vi "FetchAllDbl.vi"(8 "error in (no error)":errorcluster, 11 "NiDaqMx in":refnum<class "NiDaqMx.lvclass">) -> (0 "error out":errorcluster, 3 "NiDaqMx out":refnum<class "NiDaqMx.lvclass">)   [LabVIEW 2018, in "DigitizerPlugins.lvlib" / "NiDaqMx.lvclass"]
uses:
  NiDaqMx.lvclass
  F:/Projects/ICDAS/NistPluggableModules/Digitizer/DigitizerPlugins/DigitizerBaseClass/DigitizerBase.lvclass
  DigitizerBaseClass/DigitizerBase.lvclass/DigitizerBase.ctl
  NiDaqMx.lvclass/NiDaqMx.ctl
  DigitizerBaseClass/Typedefs/WfrmAttributes.ctl
  Accessors/Write Started.vi
  <vilib>/DAQmx/read.llb/DAQmx Read (Analog 1D Wfm NChan NSamp).vi
  DigitizerBaseClass/Accessors/Read Waveforms.vi
  DigitizerBaseClass/Accessors/Write InstRef.vi
  DigitizerBaseClass/Accessors/Write Waveforms.vi
  DigitizerBaseClass/Accessors/Read InstRef.vi
  Accessors/Read Started.vi
  DigitizerBaseClass/Accessors/Read Acquisition.vi
  DigitizerBaseClass/Accessors/Read SyncInfo.vi
  Accessors/Read TsQue.vi
  <vilib>/DAQmx/miscellaneous.llb/DAQmx Fill In Error Info.vi
  DigitizerBaseClass/DigitizerBase.lvclass
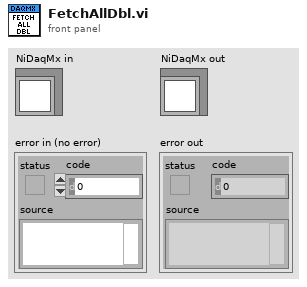
[diagram p1: front panel]
types:
  T1 = typedef "DigitizerPlugins.lvlib/DigitizerBase.lvclass/WfrmAttributes.ctl" = cluster{"XOffset":dbl, "ActualPts":i64, "FirstValid":i64}
  T2 = typedef "DigitizerPlugins.lvlib/DigitizerBase.lvclass/Acquisition.ctl" = cluster{"SampleRate":dbl, "RecordSize":i32, "NumRecords":i32, "SampleMode":i32, "Timeout (ms)":i32}
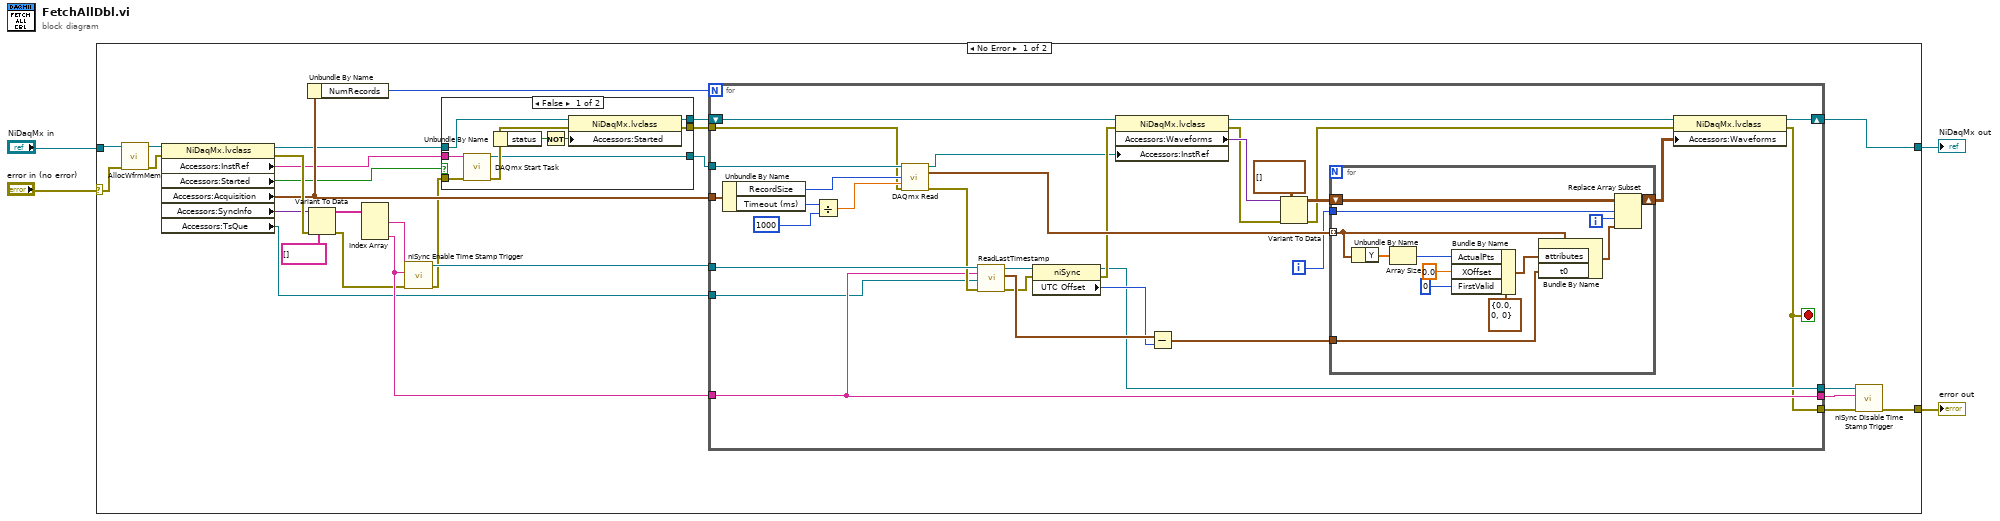
[diagram p0: block diagram]
diagram:
  n1 = case shown="No Error" "error in (no error)" {
    selector: "error in (no error)" -> [w30 w89]
    tunnel: [w15 w89] -> w3
    tunnel: [w31 w88] -> w1
    tunnel: "NiDaqMx in" -> [w29 w88]
    frame No Error {
      n2 = call-dynamic "AllocWfrmMem.vi"("error in (no error)"=w30, "DigitizerBase in"=w29) -> ("error out"=w27:errorcluster, "DigitizerBase out"=w28:refnum<class "NiDaqMx.lvclass">)  [unwired: 8 in]
      n3 = property class="NiDaqMx.lvclass"(reference=w28, error in=w27) -> (reference out=w10:refnum<class "NiDaqMx.lvclass">, error out=w25:errorcluster, "Accessors:InstRef"=w7:string, "Accessors:Started"=w8:bool, "Accessors:Acquisition"=w12:T2, "Accessors:SyncInfo"=w13:variant, "Accessors:TsQue"=w14:refnum<queue>)
      n4 = Unbundle By Name(w12) -> ("NumRecords"=w26:i32)
      n5 = Variant To Data(error in=w25, type=string[] [], Variant=w13) -> (data=w23:string[], error out=w19:errorcluster)
      n6 = Index Array(array=w23) -> (element #1=w21:string, element #3=w20:string)  [unwired: 3 in, 1 out]
      n7 = call <instrlib>:"niSync Enable Time Stamp Trigger.vi"("error in (no error)"=w19, "terminal"=w20, "instrument handle"=w21) -> ("error out"=w11:errorcluster, "instrument handle out"=w22:refnum<k15>)  [unwired: 6 in]
      n8 = case shown="False" w8 {
        tunnel: w11 -> [w40 w42]
        tunnel: w10 -> [w39 w43]
        tunnel: [w35 w43] -> w9
        tunnel: [w34 w42] -> w5
        tunnel: w7 -> [w33 w41]
        tunnel: [w32 w41] -> w6
        frame False {
          n9 = call <vilib>:"DAQmx Start Task.vi"("task/channels in"=w33, "error in"=w40) -> ("task out"=w32:refnum<k21>, "error out"=w36:errorcluster)  [unwired: 12 in]
          n10 = Unbundle By Name(w36) -> ("status"=w38:bool)
          n11 = Not(x=w38) -> (.not. x?=w37:bool)
          n12 = property class="NiDaqMx.lvclass"(reference=w39, error in=w36, "Accessors:Started"=w37) -> (reference out=w35:refnum<class "NiDaqMx.lvclass">, error out=w34:errorcluster)
        }
        frame True {
        }
      }
      n13 = for {
        N: w26 -> [_]
        tunnel: w6 -> [w72]
        tunnel: w12 -> [w66]
        shift-right: [w67] -> w31
        shift-left: w9 -> [w68]
        tunnel: w22 -> [w57]
        tunnel: w20 -> [w49]
        tunnel: [w49] -> w17
        tunnel: [w48] -> w18
        tunnel: [w47] -> w16
        tunnel: w14 -> [w46]
        tunnel: w5 -> [w45]
        i -> [w60]
        stop <- w47 stop-if-true
        n14 = Unbundle By Name(w66) -> ("RecordSize"=w71:i32, "Timeout (ms)"=w74:i32)
        n15 = Divide(x=w74, y=1000) -> (x/y=w70:dbl)
        n16 = call-poly <vilib>:"DAQmx Read.vi"("task/channels in"=w72, "number of samples per channel"=w71, "timeout"=w70, "error in"=w45) -> ("task out"=w44:refnum<k21>, "data"=w69:waveform(dbl)[], "error out"=w56:errorcluster)  [unwired: 9 in]
        n17 = call "ReadLastTimestamp.vi"("error in (no error)"=w56, "TsQue"=w46, "Terminal"=w49, "instrument handle"=w57) -> ("error out"=w51:errorcluster, "time stamp out"=w55:timestamp, "instrument handle out"=w52:refnum<k15>)  [unwired: 5 in]
        n18 = property class="niSync"(reference=w52, error in=w51) -> (reference out=w48:refnum<k15>, error out=w50:errorcluster, "UTC Offset"=w54:i32)
        n19 = property class="NiDaqMx.lvclass"(reference=w68, error in=w50, "Accessors:InstRef"=w44) -> (reference out=w65:refnum<class "NiDaqMx.lvclass">, error out=w62:errorcluster, "Accessors:Waveforms"=w63:variant)
        n20 = Subtract(x=w55, y=w54) -> (x-y=w53:timestamp)
        n21 = Variant To Data(error in=w62, type=waveform(dbl)[][] [], Variant=w63) -> (data=w61:waveform(dbl)[][], error out=w59:errorcluster)
        n22 = for {
          tunnel: w69 -> [w85] mode=indexing
          shift-right: [w79] -> w58
          shift-left: w61 -> [w80]
          tunnel: w60 -> [w76]
          tunnel: w53 -> [w75]
          i -> [w77]
          n23 = Unbundle By Name(w85) -> ("Y"=w83:dbl[])
          n24 = Array Size(array=w83) -> (size(s)=w84:i32)
          n25 = Bundle By Name(cluster=T1 {"XOffset"=0.0, "ActualPts"=0, "FirstValid"=0} ("Attributes"), "ActualPts"=w84, "XOffset"=0.0, "FirstValid"=i64 0) -> (w86:T1)
          n26 = Bundle By Name(cluster=w85, "attributes"=w86, "t0"=w75) -> (w78:waveform(dbl))
          n27 = Replace Array Subset(array=w80, new element=w78, index (row)=w76, index (col)=w77) -> (w79:waveform(dbl)[][])
        }
        n28 = property class="NiDaqMx.lvclass"(reference=w65, error in=w59, "Accessors:Waveforms"=w58) -> (reference out=w67:refnum<class "NiDaqMx.lvclass">, error out=w47:errorcluster)
      }
      n29 = call <instrlib>:"niSync Disable Time Stamp Trigger.vi"("error in (no error)"=w16, "terminal"=w17, "instrument handle"=w18) -> ("error out"=w15:errorcluster)  [unwired: 6 in, 1 out]
    }
    frame Error {
    }
  }
  "error out" <- w3
  "NiDaqMx out" <- w1
